vi "Calibra.vi"() -> (1 "SurtOk?":bool, 2 "Factor Potència Out":dbl)   [LabVIEW 2017]
uses:
  <vilib>/registry/registry.llb/Registry RtKey.ctl
  <vilib>/registry/registry.llb/Registry View.ctl
  <vilib>/registry/registry.llb/Write Registry Value Simple STR.vi
panel:
  in  "Factor Potència":dbl
  in  "Nom Sensor Temperatura":string
  in  "error in (no error)":errorcluster
  in  "Cancel":bool
  in  "OK Button":bool
  out "error out":errorcluster
  in  "Pendent Temp_1":dbl
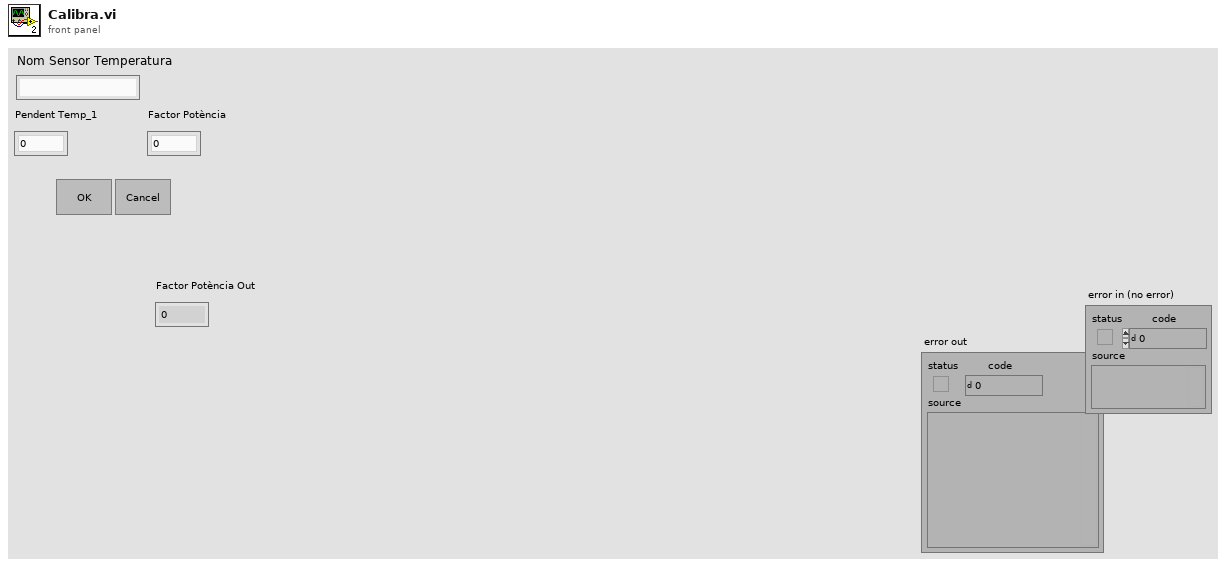
[diagram p1: front panel]
types:
  T1 = typedef "Registry RtKey.ctl" = enum32{"HKEY_CLASSES_ROOT", "HKEY_CURRENT_USER", "HKEY_LOCAL_MACHINE", "HKEY_USERS", "HKEY_PERFORMANCE_DATA", "HKEY_CURRENT_CONFIG", "HKEY_DYN_DATA"}
  T2 = typedef "Registry View.ctl" = u16
  T3 = typedef "Registry refnum.ctl" = refnum<k1>
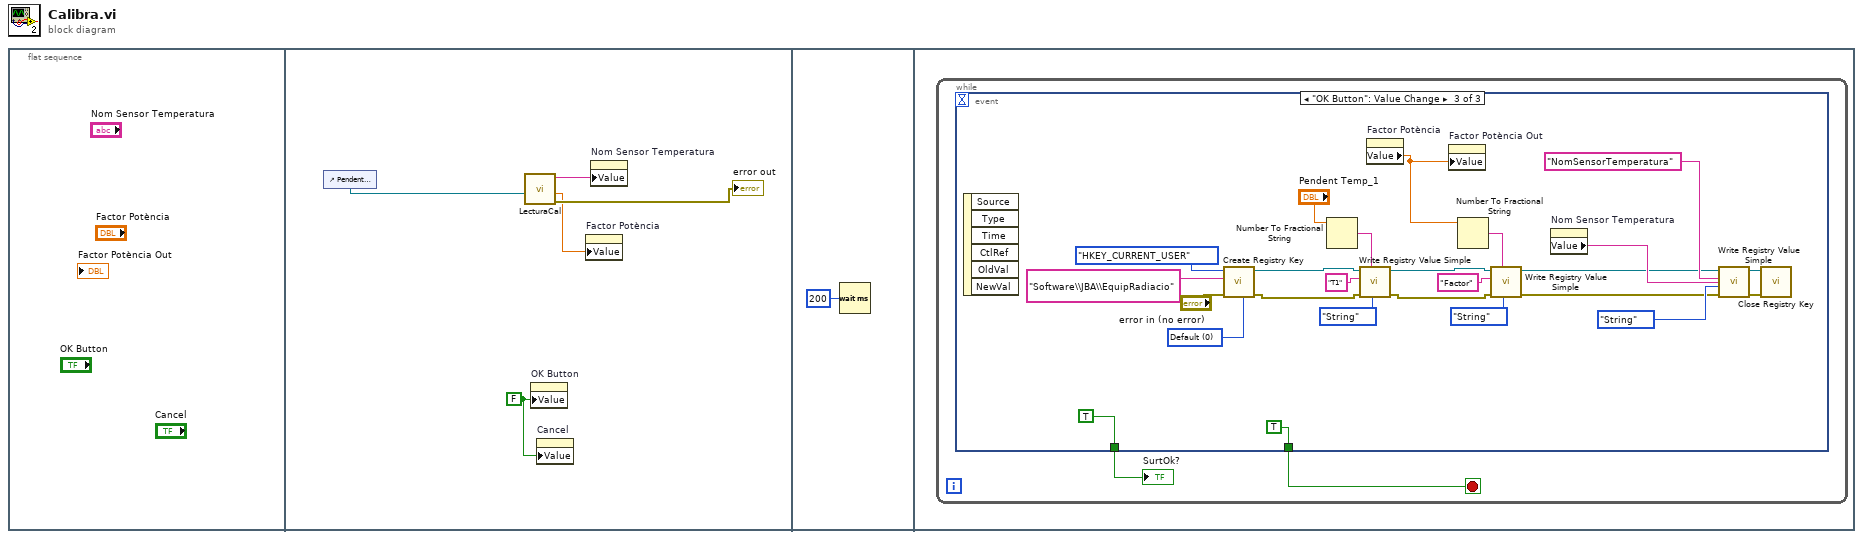
[diagram p0: block diagram]
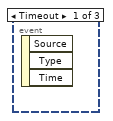
[diagram p2: hidden frame]
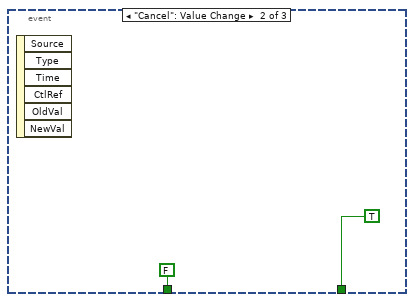
[diagram p3: hidden frame]
diagram:
  n1 = flat-sequence {
    frame #0 {
    }
    frame #1 {
      w3 = FALSE ("OK Button")
      n2 = control-ref of="Pendent Temp_1"() -> (w5:refnum<vi>)
      n3 = call "LecturaCal.vi"("T1"=w5) -> ("error out"=→"error out":errorcluster, "Factor Potència"=w1:dbl, "Nom Sensor Temperatura"=w2:string)  [unwired: 8 in]
      n4 = property on="OK Button" class="Bool (strict)"("Value"=w3) -> ()  [unwired: 2 in, 2 out]
      n5 = property on="Cancel" class="Bool (strict)"("Value"=w3) -> ()  [unwired: 2 in, 2 out]
      n6 = property on="Factor Potència" class="DigNum (strict)"("Value"=w1) -> ()  [unwired: 2 in, 2 out]
      n7 = property on="Nom Sensor Temperatura" class="Str"("Value"=w2) -> ()  [unwired: 2 in, 2 out]
    }
    frame #2 {
      n8 = Wait (ms)(milliseconds to wait=u32 200) -> ()  [unwired: 1 out]
    }
    frame #3 {
      n9 = while {
        stop <- w8 stop-if-true
        n10 = event shown="[2] \"OK Button\": Value Change" {
          selector: _ -> [_ _ _]
          dyn-events: _ -> [_ _ _]
          timeout: _ -> [_ _ _]
          tunnel: [_ TRUE TRUE ("Ok?")] -> w8
          tunnel: [_ FALSE TRUE] -> w7
          event Timeout {
            n11 = event-data() -> ()  [unwired: 1 in, 3 out]
          }
          event "Cancel": Value Change {
            n12 = event-data() -> ()  [unwired: 1 in, 6 out]
          }
          event "OK Button": Value Change {
            w32 = T2 0 items=["Default"=0, "KEY_WOW64_64KEY"=8, "KEY_WOW64_32KEY"=9] ("registry view")
            n13 = event-data() -> ()  [unwired: 1 in, 6 out]
            n14 = call <vilib>:"Create Registry Key.vi"("registry view"=w32, "error in (no error)"="error in (no error)", "subkey"="Software\\JBA\\EquipRadiacio", "root key (HKEY_LOCAL_MACHINE)"=Registry_RtKey."HKEY_CURRENT_USER") -> ("error out"=w20:errorcluster, "refnum out"=w21:T3)  [unwired: 5 in, 1 out]
            n15 = Number To Fractional String(number="Pendent Temp_1") -> (F-format string=w28:string)  [unwired: 3 in]
            n16 = call-poly <vilib>:"Write Registry Value Simple.vi"("String/Binary data"=w28, "error in (no error)"=w20, "simple data type"=enum16{"String", "Binary", "DWORD"}."String", "value"="T1", "refnum"=w21) -> ("error out"=w14:errorcluster, "refnum out"=w15:T3)  [unwired: 3 in]
            n17 = property on="Factor Potència" class="DigNum (strict)"() -> ("Value"=w11:dbl)  [unwired: 2 in, 2 out]
            n18 = property on="Factor Potència Out" class="DigNum (strict)"("Value"=w11) -> ()  [unwired: 2 in, 2 out]
            n19 = Number To Fractional String(number=w11) -> (F-format string=w16:string)  [unwired: 3 in]
            n20 = call-poly <vilib>:"Write Registry Value Simple.vi"("String/Binary data"=w16, "error in (no error)"=w14, "simple data type"=enum16{"String", "Binary", "DWORD"}."String", "value"="Factor", "refnum"=w15) -> ("error out"=w12:errorcluster, "refnum out"=w13:T3)  [unwired: 3 in]
            n21 = property on="Nom Sensor Temperatura" class="Str"() -> ("Value"=w23:string)  [unwired: 2 in, 2 out]
            n22 = call-poly <vilib>:"Write Registry Value Simple.vi"("String/Binary data"=w23, "error in (no error)"=w12, "simple data type"=enum16{"String", "Binary", "DWORD"}."String", "value"="NomSensorTemperatura", "refnum"=w13) -> ("error out"=w24:errorcluster, "refnum out"=w25:T3)  [unwired: 3 in]
            n23 = call <vilib>:"Close Registry Key.vi"("error in (no error)"=w24, "refnum"=w25) -> ()  [unwired: 5 in, 1 out]
          }
        }
        "SurtOk?" <- w7
      }
    }
  }
